vi "Initialize_Button_Interrupt.vi"(8 "error in (no error)":errorcluster) -> (0 "error out":errorcluster, 2 "Event Registration Refnum 2":refnum<event-registration>, 3 "Button Events":T1)   [LabVIEW 2014]
uses:
  <userlib>/UCSD Robotics Lab/Robotics-Cape/LV/libroboticscape.lvlib
  rc_interrupt/LV/Interrupt.lvlib
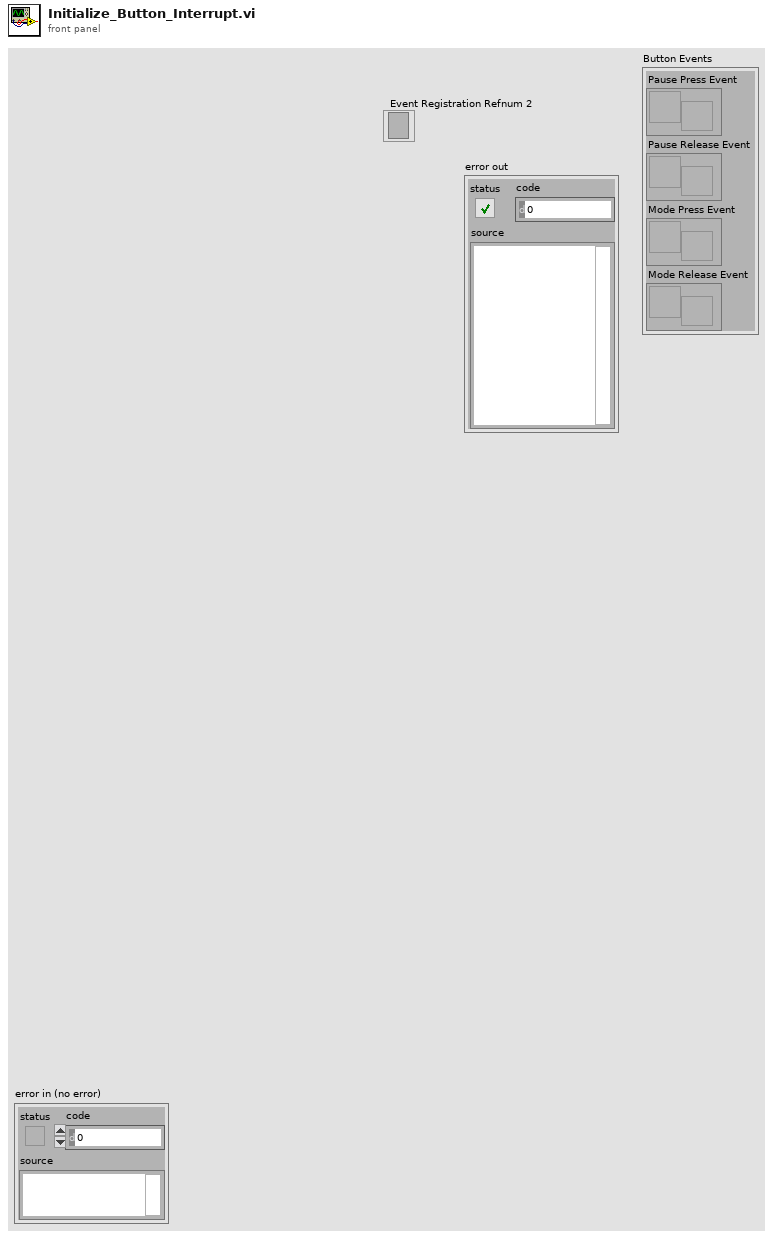
[diagram p1: front panel]
types:
  T1 = cluster{"Pause Press Event":refnum<user-event>, "Pause Release Event":refnum<user-event>, "Mode Press Event":refnum<user-event>, "Mode Release Event":refnum<user-event>}
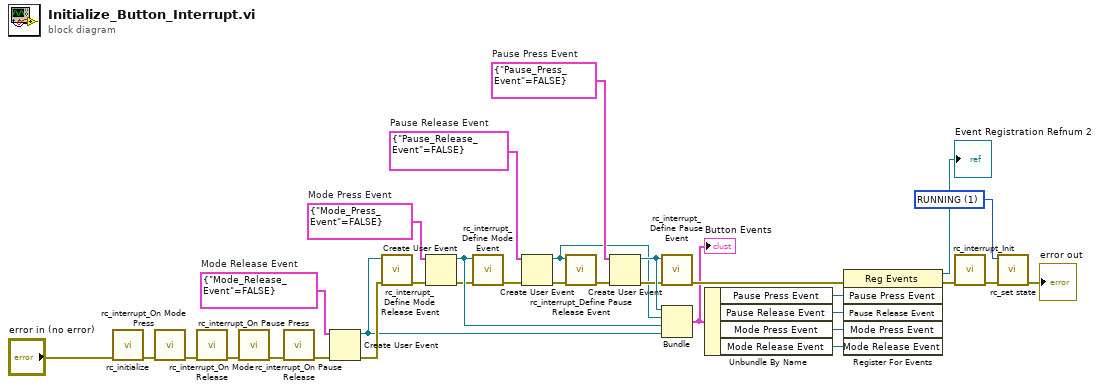
[diagram p0: block diagram]
diagram:
  w6 = cluster{"Pause_Release_Event":bool} {"Pause_Release_Event"=FALSE}  # Pause Release Event
  w26 = cluster{"Mode_Press_Event":bool} {"Mode_Press_Event"=FALSE}  # Mode Press Event
  w25 = cluster{"Mode_Release_Event":bool} {"Mode_Release_Event"=FALSE}  # Mode Release Event
  w27 = u32 1 items=["UNINITIALIZED", "RUNNING", "PAUSED", "EXITING"] ("new_state")
  w32 = cluster{"Pause_Press_Event":bool} {"Pause_Press_Event"=FALSE}  # Pause Press Event
  n1 = call <userlib>:"rc_initialize.vi"("error in (no error)"="error in (no error)") -> ("error out"=w20:errorcluster)  [unwired: 9 in, 1 out]
  n2 = call "rc_interrupt_On Mode Press.vi"("error in (no error)"=w20) -> ("error out"=w2:errorcluster)  [unwired: 9 in, 1 out]
  n3 = call "rc_interrupt_On Mode Release.vi"("error in (no error)"=w2) -> ("error out"=w1:errorcluster)  [unwired: 9 in, 1 out]
  n4 = call "rc_interrupt_On Pause Press.vi"("error in (no error)"=w1) -> ("error out"=w19:errorcluster)  [unwired: 9 in, 1 out]
  n5 = call "rc_interrupt_On Pause Release.vi"("error in (no error)"=w19) -> ("error out"=w18:errorcluster)  [unwired: 9 in, 1 out]
  n6 = Create User Event(user event datatype=w25, error in=w18) -> (user event=w16:refnum<user-event>, error out=w17:errorcluster)
  n7 = call "rc_interrupt_Define Mode Release Event.vi"("error in (no error)"=w17, "user event in"=w16) -> ("error out"=w15:errorcluster)  [unwired: 8 in, 1 out]
  n8 = Create User Event(user event datatype=w26, error in=w15) -> (user event=w14:refnum<user-event>, error out=w13:errorcluster)
  n9 = call "rc_interrupt_Define Mode Event.vi"("error in (no error)"=w13, "user event in"=w14) -> ("error out"=w8:errorcluster)  [unwired: 8 in, 1 out]
  n10 = Create User Event(user event datatype=w6, error in=w8) -> (user event=w5:refnum<user-event>, error out=w7:errorcluster)
  n11 = call "rc_interrupt_Define Pause Release Event.vi"("error in (no error)"=w7, "user event in"=w5) -> ("error out"=w12:errorcluster)  [unwired: 8 in, 1 out]
  n12 = Create User Event(user event datatype=w32, error in=w12) -> (user event=w11:refnum<user-event>, error out=w10:errorcluster)
  n13 = call "rc_interrupt_Define Pause Event.vi"("error in (no error)"=w10, "user event in"=w11) -> ("error out"=w9:errorcluster)  [unwired: 8 in, 1 out]
  n14 = Bundle("Pause Press Event"=w11, "Pause Release Event"=w5, "Mode Press Event"=w14, "Mode Release Event"=w16) -> (w3:T1)  [unwired: 1 in]
  "Button Events" <- w3
  n15 = Unbundle By Name(w3) -> ("Pause Press Event"=w24:refnum<user-event>, "Pause Release Event"=w23:refnum<user-event>, "Mode Press Event"=w22:refnum<user-event>, "Mode Release Event"=w21:refnum<user-event>)
  n16 = register-events(error in=w9, w24, w23, w22, w21) -> (reference out=→"Event Registration Refnum 2":refnum<event-registration>, error out=w31:errorcluster)  [unwired: 1 in]
  n17 = call "rc_interrupt_Init.vi"("error in (no error)"=w31) -> ("error out"=w29:errorcluster)  [unwired: 9 in, 1 out]
  n18 = call <userlib>:"rc_set state.vi"("error in (no error)"=w29, "new_state"=w27) -> ("error out"=→"error out":errorcluster)  [unwired: 8 in, 1 out]
